vi "AVS_SetDigOut.vi"(0 "a_hDevice":i32, 7 "a_PortId":u8, 11 "a_Status":u8) -> (4 "Output Value":i32)   [LabVIEW 2016]
uses:
  Downloads/LinuxAPIselected/RedHat/libavs.so
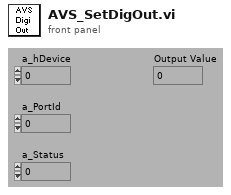
[diagram p1: front panel]
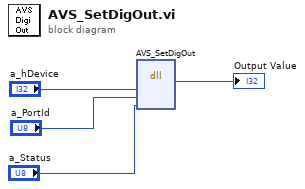
[diagram p0: block diagram]
diagram:
  n1 = dll-call lib="home/harini/Downloads/LinuxAPIselected/RedHat/libavs.so" fn="AVS_SetDigOut"("a_hDevice"="a_hDevice", "a_PortId"="a_PortId", "a_Status"="a_Status") -> ("return type"=→"Output Value":i32)  [unwired: 6 in, 2 out]
